vi "Frequency Error Update.vi"(9 "Source":dbl format="%#_13g", 11 "Target":refnum<vi>) -> ()   [LabVIEW 2018]
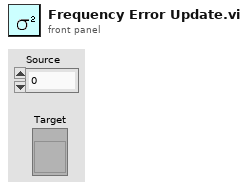
[diagram p1: front panel]
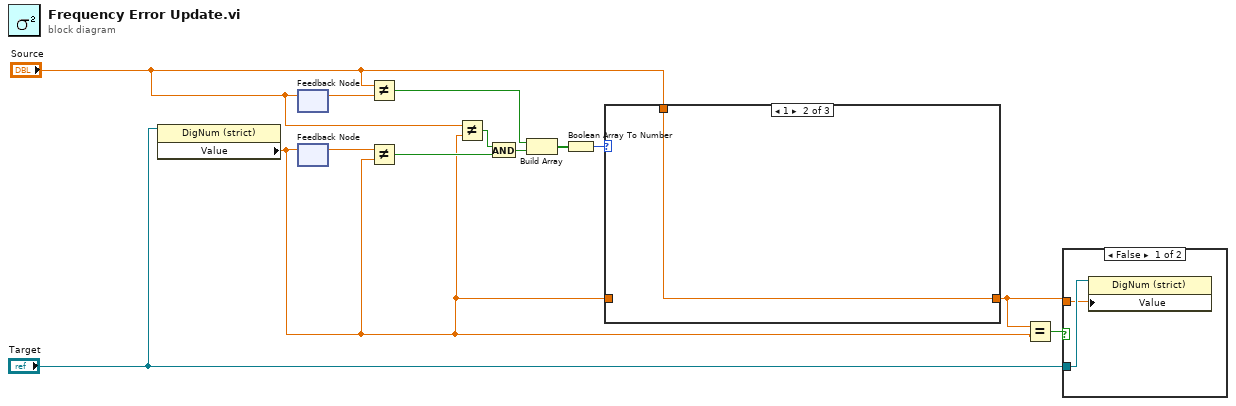
[diagram p0: block diagram]
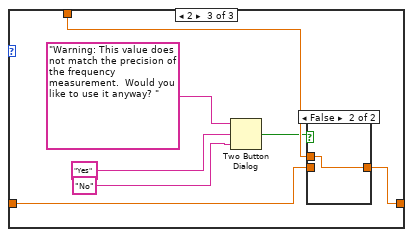
[diagram p4: hidden frame]
diagram:
  n1 = property class="DigNum (strict)"(reference="Target") -> ("Value"=w3:dbl)  [unwired: 1 in, 2 out]
  n2 = feedback #1() -> (w4:dbl)  [unwired: 1 in]
  n3 = feedback-in #1("Source") -> ()
  n4 = feedback #2() -> (w5:dbl)  [unwired: 1 in]
  n5 = feedback-in #2(w3) -> ()
  n6 = Not Equal?(x="Source", y=w4) -> (x != y?=w11:bool)
  n7 = Not Equal?(x=w5, y=w3) -> (x != y?=w10:bool)
  n8 = Not Equal?(x="Source", y=w3) -> (x != y?=w6:bool)
  n9 = And(x=w6, y=w10) -> (x .and. y?=w7:bool)
  n10 = Build Array(w11, w7) -> (w9:bool[])
  n11 = Boolean Array To Number(Boolean array=w9) -> (number=w8:u32)
  n12 = case shown="1" w8 {
    tunnel: "Source" -> [_ w15 w20]
    tunnel: w3 -> [w14 _ w22]
    tunnel: [w14 w15 w21] -> w1
    frame 0, Default {
    }
    frame 1 {
    }
    frame 2 {
      n13 = Two Button Dialog(message="Warning: This value does not match the precision of the frequency measurement.  Would you like to use it anyway? ", 1:"No", 2:"Yes") -> (T button?=w16:bool)
      n14 = case shown="False" w16 {
        tunnel: w22 -> [w23 _]
        tunnel: w20 -> [_ w24]
        tunnel: [w23 w24] -> w21
        frame True {
        }
        frame False {
        }
      }
    }
  }
  n15 = Equal?(x=w1, y=w3) -> (x = y?=w2:bool)
  n16 = case shown="False" w2 {
    tunnel: w1 -> [w25 _]
    tunnel: "Target" -> [w26 _]
    frame False {
      n17 = property class="DigNum (strict)"(reference=w26, "Value"=w25) -> ()  [unwired: 1 in, 2 out]
    }
    frame True {
    }
  }
